vi "ni579x Open.vi"(0 "fpga ref":refnum<k20>, 7 "re-initialize?":bool, 9 "bus instance":u32, 11 "Error In":errorcluster) -> (4 "Register Bus (out)":refnum<class "ni579x Register Bus v1 Host.lvclass">, 15 "Error Out":errorcluster)   [LabVIEW 2015]
doc: "Opens a session to the NI-579x Configuration Design Library. Creates a session to the Register Bus Host library and initializes the CLIP.\n\n<B>Input Parameters</B>\n\n<B>fpga ref</B> A reference to an LabVIEW FPGA created using the Open FPGA VI Reference VI\n\n<B>re-initialize?</B> Whether or not to re-initialize the FAM CLIP (resets the device configuration to its defaults).\n\n<B>bus instance</B> Used if creating multiple Register Buses to the same device.\n\n<B>Output Parameters</B>\n\n<B>Register Bus (out)</B> A new Register Bus session used in all subsequent NI-579x Configuration Design Library Host VIs."
uses:
  <instrlib>/ni579x/Register Bus/v1/Host/ni579x Register Bus v1 Host.lvclass
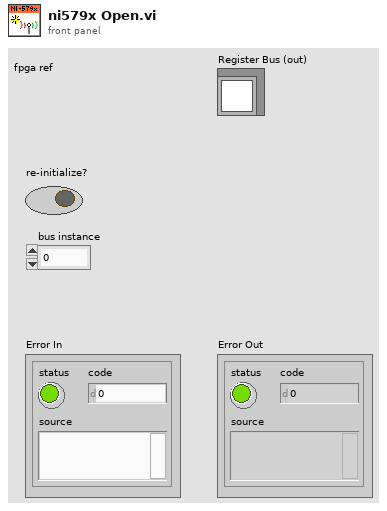
[diagram p1: front panel]
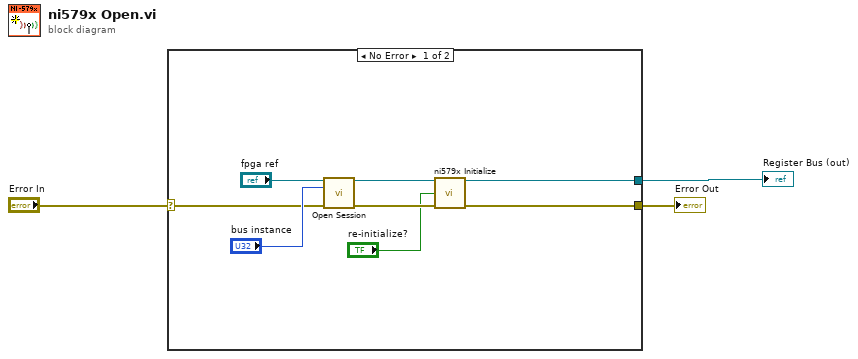
[diagram p0: block diagram]
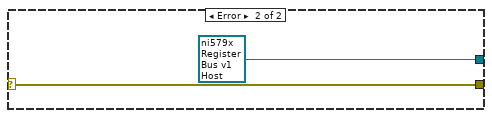
[diagram p2: hidden frame]
diagram:
  n1 = case shown="No Error" "Error In" {
    selector: "Error In" -> [w7 w13]
    tunnel: [w4 w13] -> w3
    tunnel: [w5 refnum<class "ni579x Register Bus v1 Host.lvclass"> refnum ("Register Bus (out)")] -> w1
    frame No Error {
      n2 = call <instrlib>:"Open Session.vi"("fpga ref"="fpga ref", "bus instance"="bus instance", "error in"=w7) -> ("session out"=w11:refnum<class "ni579x Register Bus v1 Host.lvclass">, "error out"=w10:errorcluster)  [unwired: 11 in]
      n3 = call <instrlib>:"ni579x Initialize.vi"("Register Bus"=w11, "re-initialize?"="re-initialize?", "Error In"=w10) -> ("Register Bus (out)"=w5:refnum<class "ni579x Register Bus v1 Host.lvclass">, "Error Out"=w4:errorcluster)  [unwired: 11 in]
    }
    frame Error {
    }
  }
  "Register Bus (out)" <- w1
  "Error Out" <- w3
